vi "select names.vi"(11 "List Selected":T2(array[cluster])) -> (3 "Names":T1)   [LabVIEW 2023]
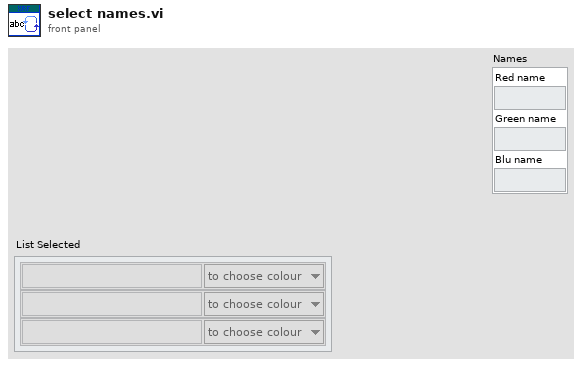
[diagram p1: front panel]
types:
  T1 = cluster{"Red name":string, "Green name":string, "Blu name":string}
  T2 = cluster{"Table":string, "color":enum16{"to choose colour", "red", "green", "blue"}}[]
  T3 = enum16{"to choose colour", "red", "green", "blue"}
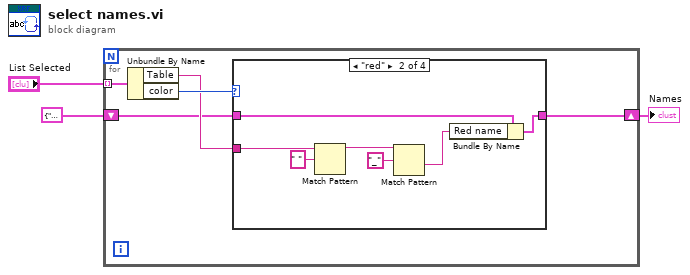
[diagram p0: block diagram]
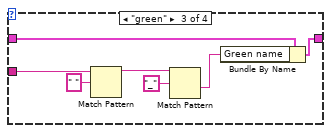
[diagram p3: hidden frame]
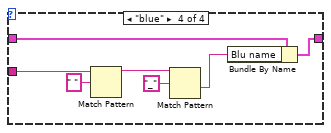
[diagram p4: hidden frame]
diagram:
  n1 = for {
    tunnel: "List Selected" -> [w8] mode=indexing
    shift-right: [w4] -> w1
    shift-left: T1 {"Red name"="", "Green name"="", "Blu name"=""} ("Names") -> [w5]
    n2 = Unbundle By Name(w8) -> ("Table"=w6:string, "color"=w7:T3)
    n3 = case shown="\"red\"" w7 {
      tunnel: w6 -> [_ w16 w23 w30]
      tunnel: w5 -> [w9 w12 w19 w26]
      tunnel: [w9 w11 w18 w25] -> w4
      frame "to choose colour", Default {
      }
      frame "red" {
        n4 = Match Pattern(string=w16, regular expression=" ") -> (before substring=w14:string)  [unwired: 1 in, 3 out]
        n5 = Match Pattern(string=w14, regular expression="_") -> (after substring=w10:string)  [unwired: 1 in, 3 out]
        n6 = Bundle By Name(cluster=w12, "Red name"=w10) -> (w11:T1)
      }
      frame "green" {
        n7 = Match Pattern(string=w23, regular expression=" ") -> (before substring=w21:string)  [unwired: 1 in, 3 out]
        n8 = Match Pattern(string=w21, regular expression="_") -> (after substring=w17:string)  [unwired: 1 in, 3 out]
        n9 = Bundle By Name(cluster=w19, "Green name"=w17) -> (w18:T1)
      }
      frame "blue" {
        n10 = Match Pattern(string=w30, regular expression=" ") -> (before substring=w28:string)  [unwired: 1 in, 3 out]
        n11 = Match Pattern(string=w28, regular expression="_") -> (after substring=w24:string)  [unwired: 1 in, 3 out]
        n12 = Bundle By Name(cluster=w26, "Blu name"=w24) -> (w25:T1)
      }
    }
  }
  "Names" <- w1
